vi "__Local List Menu Handler.vi"(7 "FileManager Data":T1, 8 "error in (no error)":errorcluster, 11 "Menuitem Tag":string) -> (0 "error out":errorcluster)   [LabVIEW 2011]
doc: "Handles the Local list right-click menu."
uses:
  __File manager Data type.ctl
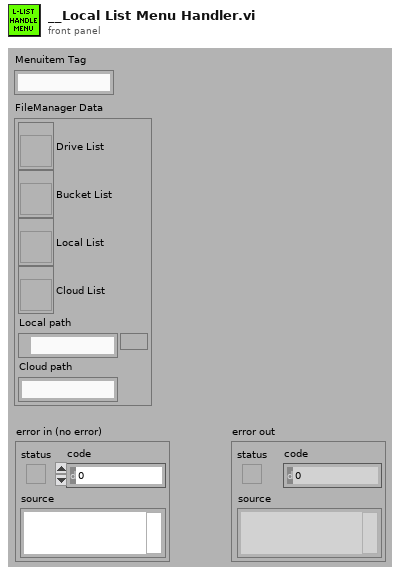
[diagram p1: front panel]
types:
  T1 = typedef "__File manager Data type.ctl" = cluster{"Drive List":refnum<vi>, "Bucket List":refnum<vi>, "Local List":refnum<vi>, "Cloud List":refnum<vi>, "Local path":path, "Cloud path":string}
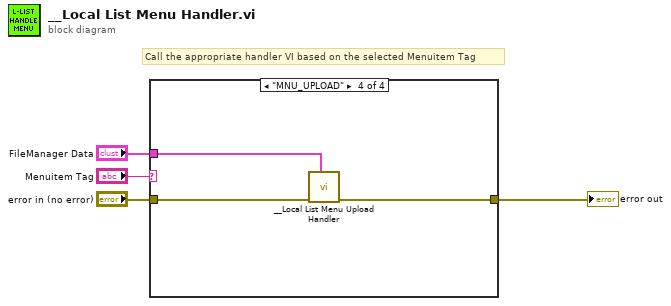
[diagram p0: block diagram]
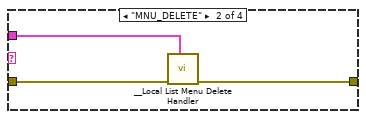
[diagram p3: hidden frame]
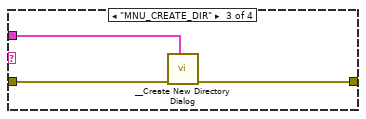
[diagram p4: hidden frame]
diagram:
  # "Call the appropriate handler VI based on the selected Menuitem Tag"
  n1 = case shown="\"MNU_UPLOAD\"" "Menuitem Tag" {
    tunnel: "error in (no error)" -> [w5 w8 w11 w14]
    tunnel: [w5 w7 w9 w12] -> w2
    tunnel: "FileManager Data" -> [_ w6 w10 w13]
    frame Default {
    }
    frame "MNU_DELETE" {
      n2 = call "__Local List Menu Delete Handler.vi"("FileManager Data"=w6, "error in (no error)"=w8) -> ("error out"=w7:errorcluster)  [unwired: 9 in]
    }
    frame "MNU_CREATE_DIR" {
      n3 = call "__Create New Directory Dialog.vi"("FileManager Data"=w10, "error in (no error)"=w11) -> ("error out"=w9:errorcluster)  [unwired: 9 in]
    }
    frame "MNU_UPLOAD" {
      n4 = call "__Local List Menu Upload Handler.vi"("FileManager Data"=w13, "error in (no error)"=w14) -> ("error out"=w12:errorcluster)  [unwired: 9 in]
    }
  }
  "error out" <- w2
